vi "Prefrences.vi"(8 "error in":errorcluster) -> ()   [LabVIEW 2015]
uses:
  <vilib>/Rock Robotics/Network Tables/NT Read String.vi
  <vilib>/Rock Robotics/Network Tables/NT Read String Array.vi
  <vilib>/Utility/config.llb/Read Key (String).vi
  <vilib>/Rock Robotics/Network Tables/NT Write String Array.vi
  <vilib>/Utility/config.llb/Write Key (String).vi
  <vilib>/Utility/config.llb/NI_LVConfig.lvlib
panel:
  out "error out 2":errorcluster
  in  "Preferences":string[][](array[string])
  out "Key                              Value":string[][](array[string])
  out "error out":errorcluster
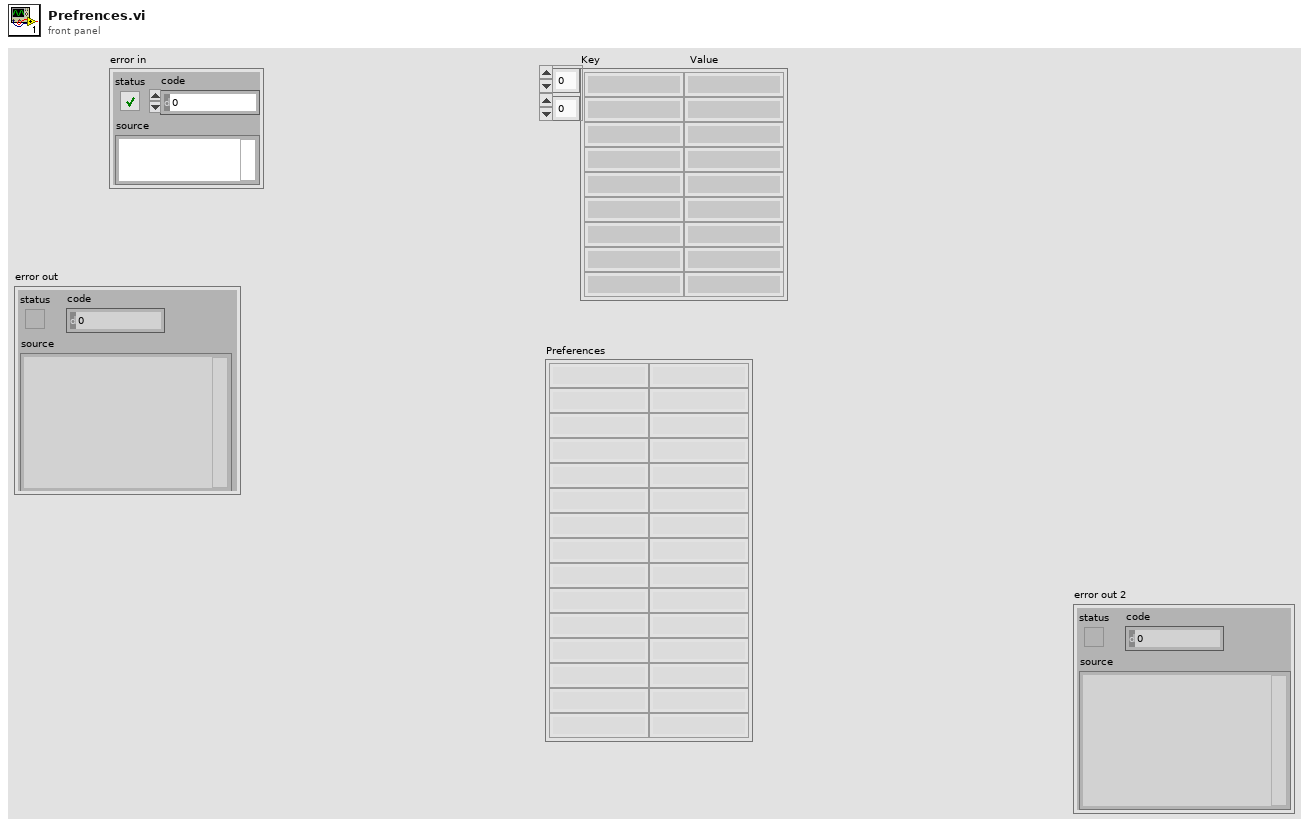
[diagram p1: front panel]
types:
  T1 = typedef "NI_LVConfig.lvlib/Config Data RefNum.ctl" = refnum<k1>
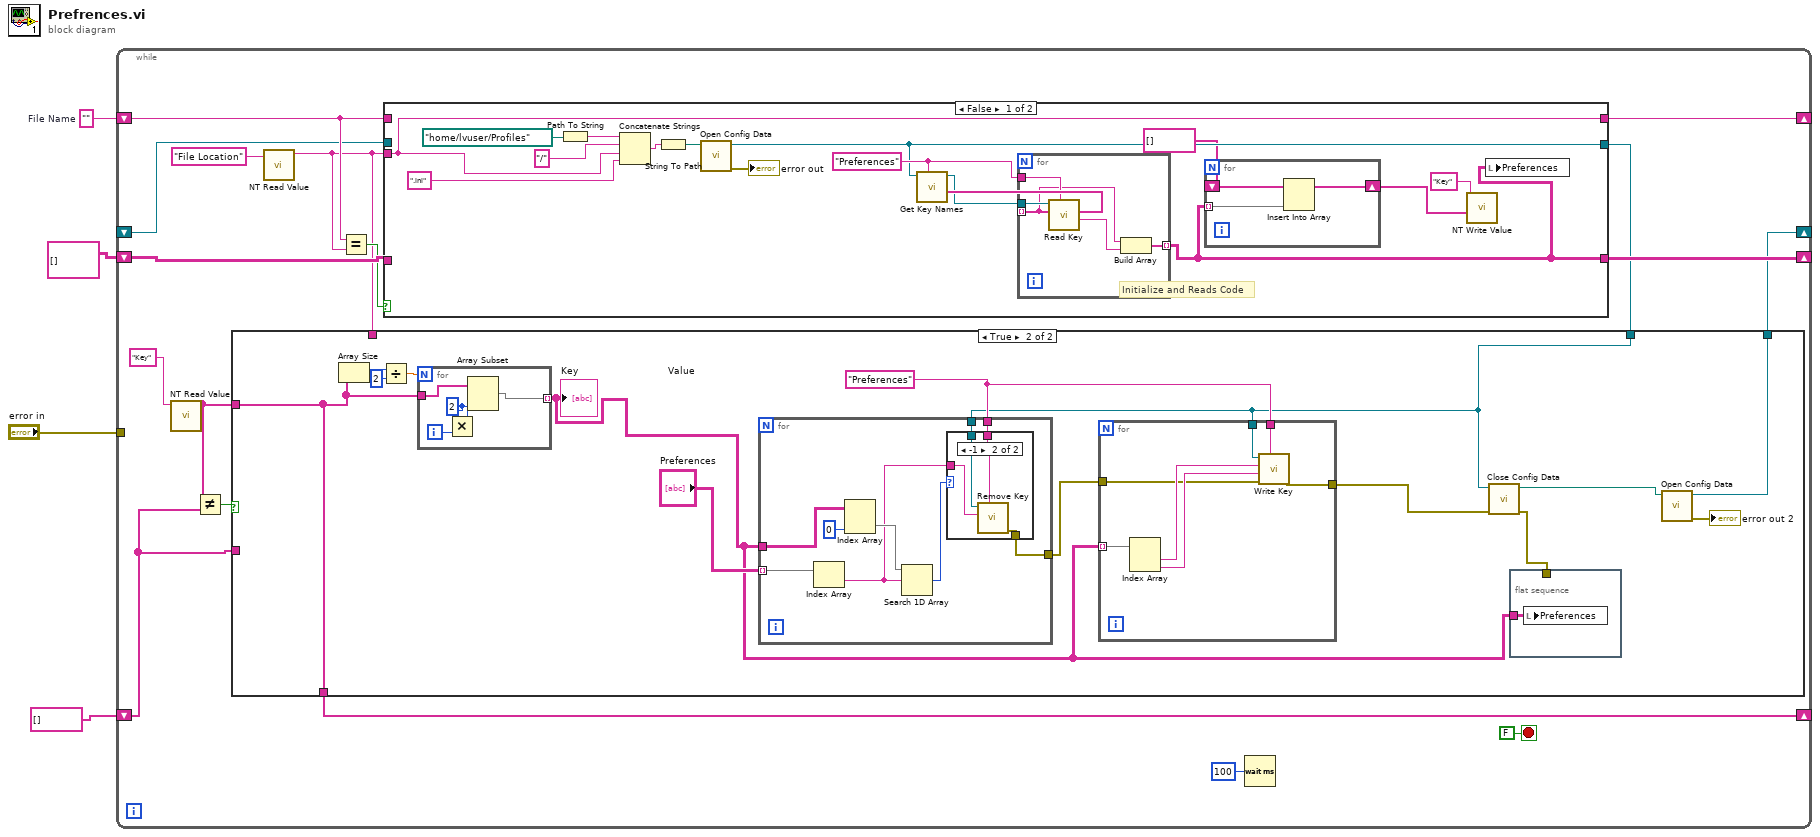
[diagram p0: block diagram]
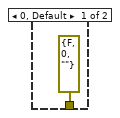
[diagram p3: hidden frame]
diagram:
  w4 = ""  # File Name
  n1 = while {
    shift-right: [w9] -> _
    shift-left: w4 -> [w17]
    shift-right: [w20] -> _
    shift-left: string[][] [] -> [w19]
    shift-right: [w6] -> _
    shift-left: _ -> [w15]
    tunnel: "error in" -> [_]
    shift-right: [w10] -> _
    shift-left: string[] [] ("String Array") -> [w11]
    stop <- FALSE stop-if-true
    n2 = call-poly <vilib>:"NT Read Value.vi"("Name"="Key") -> ("String Array"=w12:string[])  [unwired: 9 in, 1 out]
    n3 = Not Equal?(x=w12, y=w11) -> (x != y?=w13:bool)
    n4 = call-poly <vilib>:"NT Read Value.vi"("Name"="File Location") -> ("String"=w8:string)  [unwired: 9 in, 1 out]
    n5 = Equal?(x=w17, y=w8) -> (x = y?=w16:bool)
    n6 = case shown="False" w16 {
      tunnel: [w65 w91] -> w20
      tunnel: w19 -> [_ w91]
      tunnel: w8 -> [w68 _]
      tunnel: w17 -> [_ w90]
      tunnel: [w68 w90] -> w9
      tunnel: [w72 w89] -> w7
      tunnel: w15 -> [_ w89]
      frame False {
        w79 = "Preferences" ("section")
        # "Initialize and Reads Code"
        n7 = Path To String(path=path "/home/lvuser/Profiles" ("configuration file path")) -> (string=w77:string)
        n8 = Concatenate Strings(w77, "/" ("string"), w68, ".ini" ("string")) -> (w76:string)
        n9 = String To Path(string=w76) -> (path=w73:path)
        n10 = call <vilib>:"Open Config Data.vi"("configuration file path"=w73) -> ("error out"=→"error out":errorcluster, "refnum"=w72:T1)  [unwired: 8 in, 1 out]
        n11 = call <vilib>:"Get Key Names.vi"("section"=w79, "refnum"=w72) -> ("key names"=w80:string[], "refnum out"=w78:T1)  [unwired: 6 in, 2 out]
        n12 = for {
          tunnel: w80 -> [w86] mode=indexing
          tunnel: w78 -> [w88]
          tunnel: w79 -> [w87]
          tunnel: [w84] -> w65 mode=indexing
          n13 = call-poly <vilib>:"Read Key.vi"("section"=w87, "key"=w86, "refnum"=w88) -> ("value"=w85:string)  [unwired: 5 in, 3 out]
          n14 = Build Array(w86, w85) -> (w84:string[])
        }
        n15 = for {
          tunnel: w65 -> [w82] mode=indexing
          shift-right: [w81] -> w70
          shift-left: string[] [] -> [w83]
          n16 = Insert Into Array(array=w83, new element=w82) -> (w81:string[])  [unwired: 1 in]
        }
        n17 = call-poly <vilib>:"NT Write Value.vi"("String Array"=w70, "Name"="Key") -> ()  [unwired: 9 in, 1 out]
        n18 = local write "Preferences"(w65) -> ()
      }
      frame True {
      }
    }
    n19 = case shown="True" w13 {
      tunnel: w12 -> [_ w33]
      tunnel: w11 -> [w23 _]
      tunnel: [w23 w33] -> w10
      tunnel: w8 -> [_ _]
      tunnel: [w22 w30] -> w6
      tunnel: w7 -> [w22 w28]
      frame False {
      }
      frame True {
        w34 = "Preferences" ("section")
        n20 = Array Size(array=w33) -> (size(s)=w36:i32)
        n21 = Divide(x=w36, y=2) -> (x/y=w35:dbl)
        n22 = for {
          N: w35 -> [_]
          tunnel: w33 -> [w64]
          tunnel: [w63] -> w24 mode=indexing
          i -> [w62]
          w61 = 2 ("length")
          n23 = Multiply(x=w61, y=w62) -> (x*y=w60:i32)
          n24 = Array Subset(array=w64, index=w60, length=w61) -> (w63:string[])
        }
        "Key                              Value" <- w24
        n25 = for {
          tunnel: "Preferences" -> [w54] mode=indexing
          tunnel: w34 -> [w51]
          tunnel: w24 -> [w48]
          tunnel: w28 -> [w47]
          tunnel: [w46] -> w26
          n26 = Index Array(array=w54) -> (element=w50:string)  [unwired: 1 in]
          n27 = Index Array(array=w48, index (col)=0 ("disabled index (col)")) -> (element=w52:string[])  [unwired: 1 in]
          n28 = Search 1D Array(1D array=w52, element=w50) -> (index of element=w49:i32)  [unwired: 1 in]
          n29 = case shown="-1" w49 {
            tunnel: w51 -> [_ w59]
            tunnel: w50 -> [_ w58]
            tunnel: w47 -> [_ w57]
            tunnel: [errorcluster {"status"=FALSE, "code"=0, "source"=""} ("error out") w56] -> w46
            frame 0, Default {
            }
            frame -1 {
              n30 = call <vilib>:"Remove Key.vi"("section"=w59, "key"=w58, "refnum"=w57) -> ("error out"=w56:errorcluster)  [unwired: 6 in, 2 out]
            }
          }
        }
        n31 = for {
          tunnel: w24 -> [w45] mode=indexing
          tunnel: w34 -> [w44]
          tunnel: w28 -> [w41]
          tunnel: [w40] -> w27
          tunnel: w26 -> [w39]
          n32 = Index Array(array=w45) -> (element #1=w43:string, element #2=w42:string)  [unwired: 2 in]
          n33 = call-poly <vilib>:"Write Key.vi"("section"=w44, "error in (no error)"=w39, "value"=w42, "key"=w43, "refnum"=w41) -> ("error out"=w40:errorcluster)  [unwired: 4 in, 2 out]
        }
        n34 = call <vilib>:"Close Config Data.vi"("error in (no error)"=w27, "refnum"=w28) -> ("error out"=w25:errorcluster, "file path"=w29:path)  [unwired: 8 in]
        n35 = flat-sequence {
          tunnel: w25 -> [_]
          tunnel: w24 -> [w38]
          frame #0 {
            n36 = local write "Preferences"(w38) -> ()
          }
        }
        n37 = call <vilib>:"Open Config Data.vi"("configuration file path"=w29) -> ("error out"=→"error out 2":errorcluster, "refnum"=w30:T1)  [unwired: 8 in, 1 out]
      }
    }
    n38 = Wait (ms)(milliseconds to wait=u32 100) -> ()  [unwired: 1 out]
  }
